vi "Main_v2.vi"(8 "error in (no error)":errorcluster) -> (0 "error out (no error)":errorcluster)   [LabVIEW 2019]
uses:
  controls/UI_Data_v2.ctl
  support/Copy of Message Queue/All Message Queues.ctl
  support/Copy of Message Queue/Message Cluster.ctl
  controls/MetaData_v2.ctl
  support/User Event - Stop/User Event - Stop.lvlib
  support/Copy of Message Queue/Copy of Message Queue.lvlib
  support/Message Queue/Message Queue.lvlib
panel:
  out "error out":errorcluster
  in  "UI Data":T1={"Measurements"=[], "Offsets"=[], "SSC"=[], "Message Queues"={"UI"=refnum, "Acquisition"=refnum, "Logging"=refnum, "Analyze"=refnum}, "MetaData"={"Operator Name"=enum."Operator Name", "Location"=enum."Location", "Sensor SN"="Sensor SN", "Cal Tube SN"="Cal Tube SN", "Comments"="Comments"}}
  in  "Stop":bool
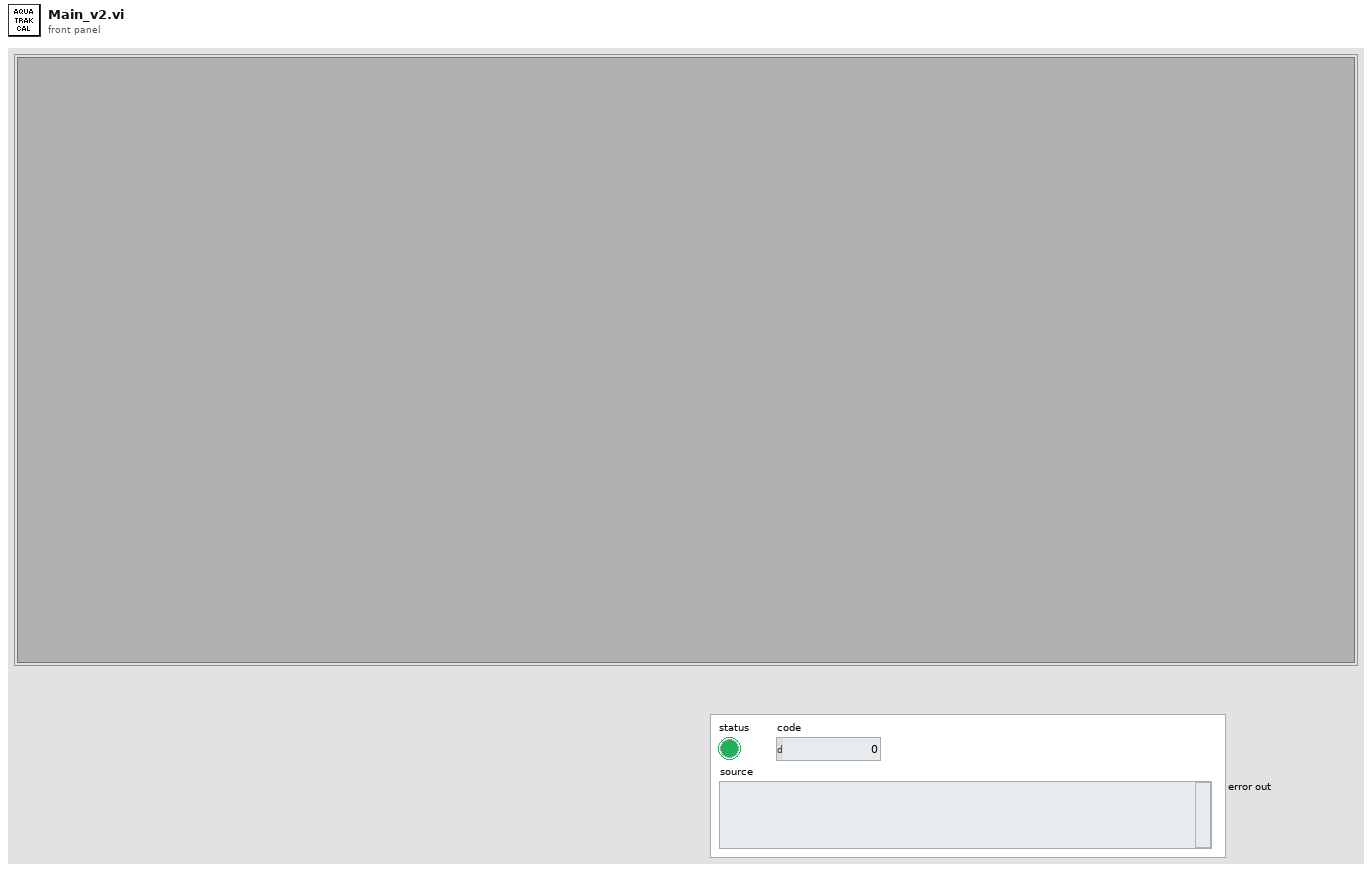
[diagram p1: front panel]
types:
  T1 = typedef "UI_Data_v2.ctl" = cluster{"Measurements":dbl[], "Offsets":dbl[], "SSC":dbl[], "Message Queues":T2, "MetaData":T3}
  T2 = typedef "Copy of Message Queue.lvlib/All Message Queues.ctl" = cluster{"UI":refnum<queue>, "Acquisition":refnum<queue>, "Logging":refnum<queue>, "Analyze":refnum<queue>}
  T3 = typedef "MetaData_v2.ctl" = cluster{"Operator Name":enum16{"Operator Name"}, "Location":enum16{"Location", "Chesapeake", "Silver Spring", "Seattle"}, "Sensor SN":string, "Cal Tube SN":string, "Comments":string}
  T4 = typedef "UserEvents_v2.ctl" = cluster{"User Event - Msg":refnum<user-event>, "User Event - Stop":refnum<user-event>}
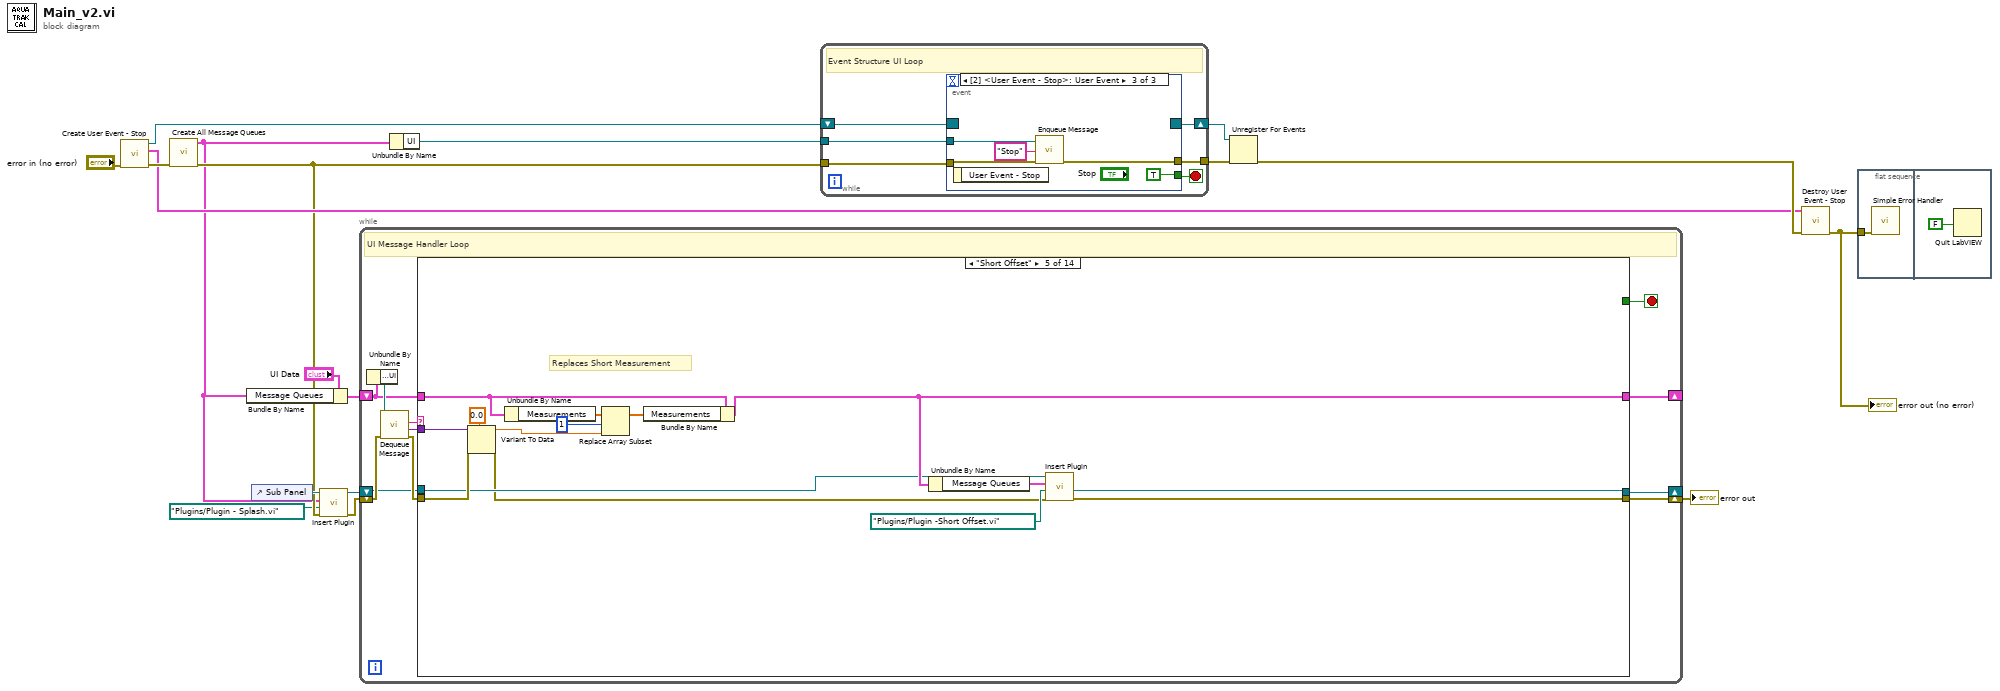
[diagram p0: block diagram]
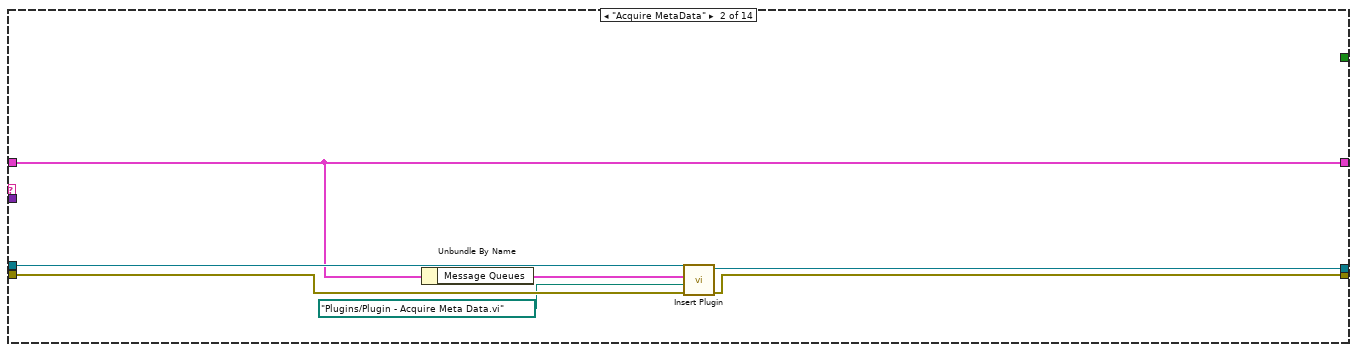
[diagram p3: hidden frame]
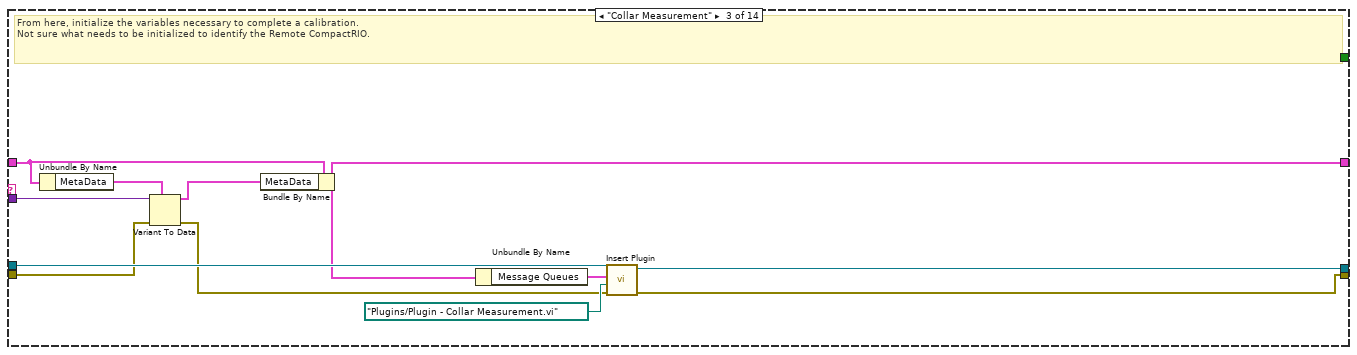
[diagram p4: hidden frame]
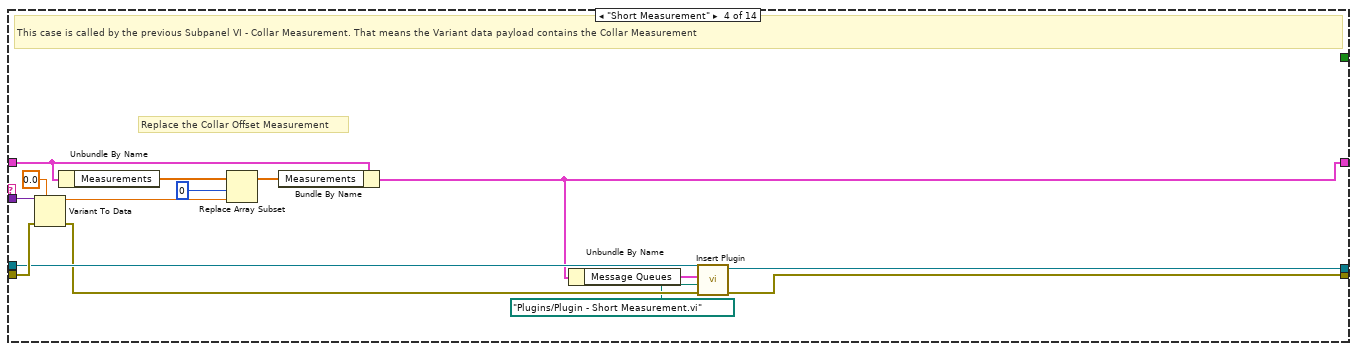
[diagram p5: hidden frame]
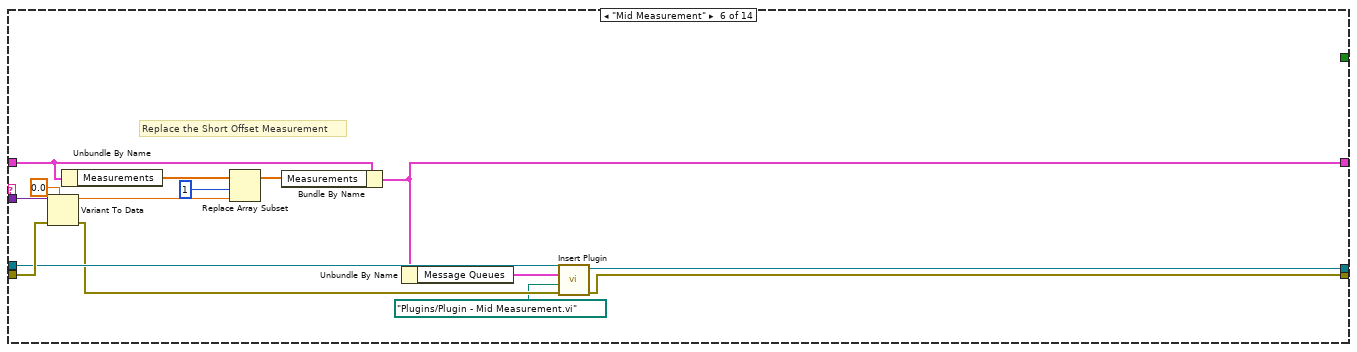
[diagram p6: hidden frame]
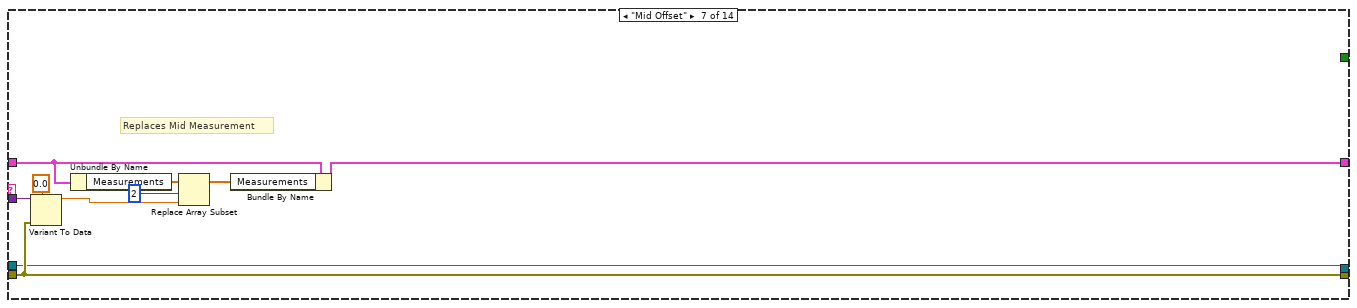
[diagram p7: hidden frame]
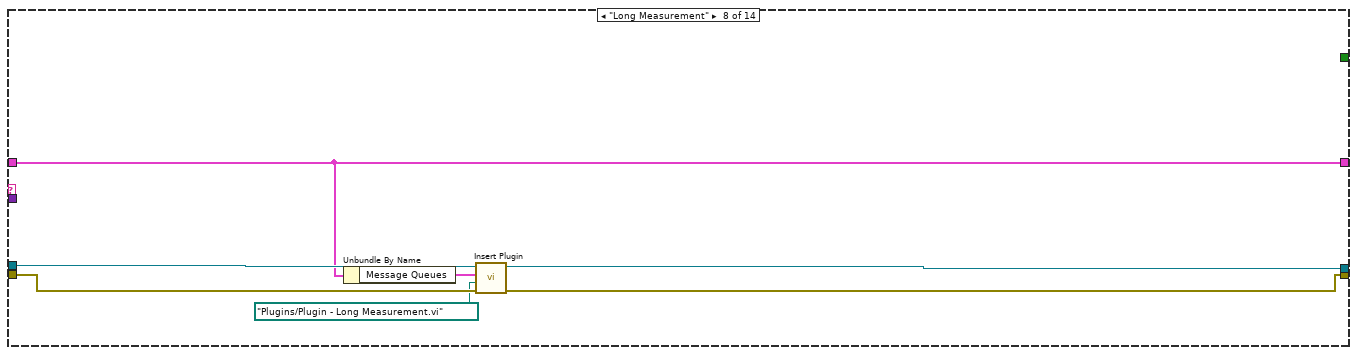
[diagram p8: hidden frame]
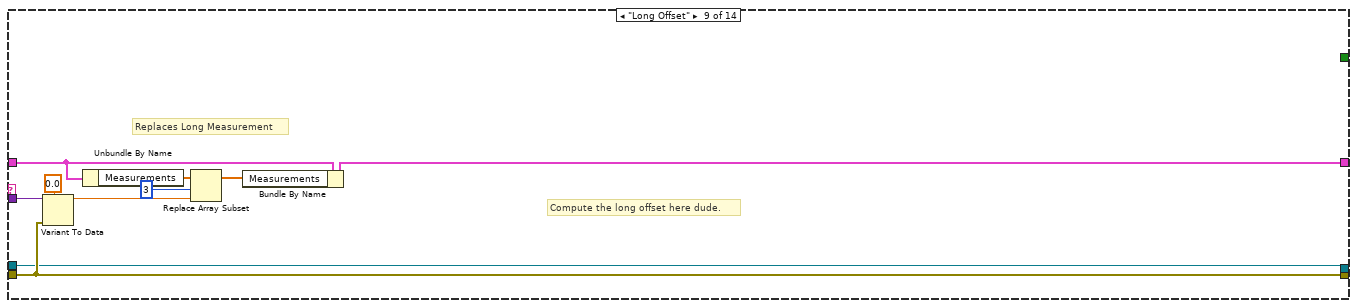
[diagram p9: hidden frame]
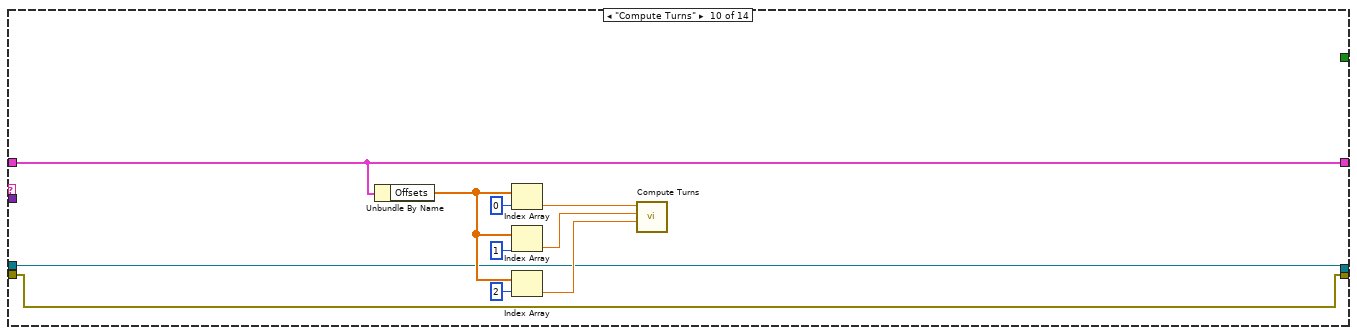
[diagram p10: hidden frame]
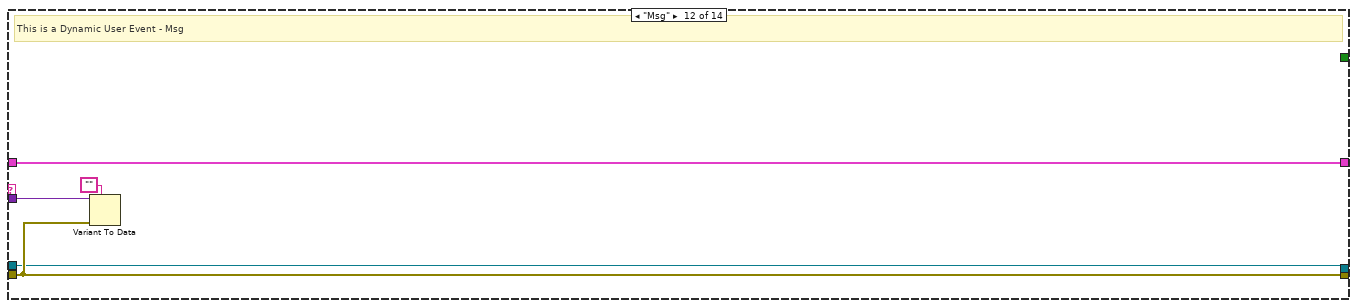
[diagram p12: hidden frame]
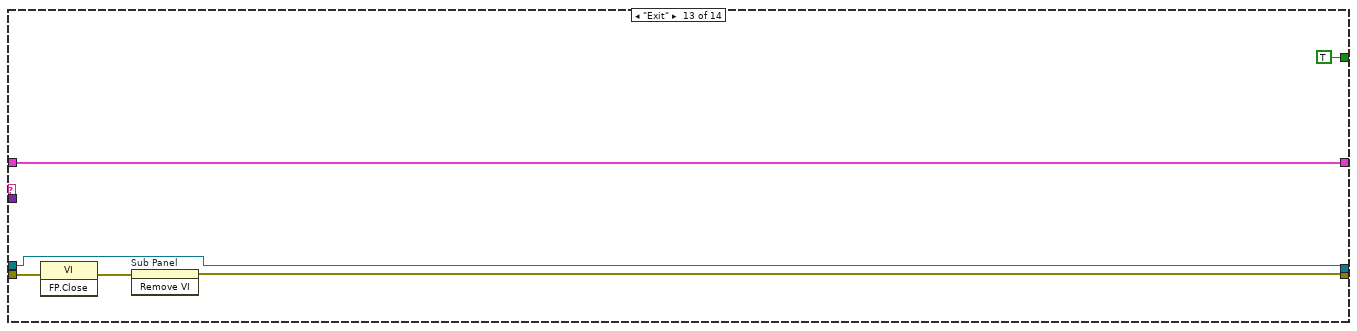
[diagram p13: hidden frame]
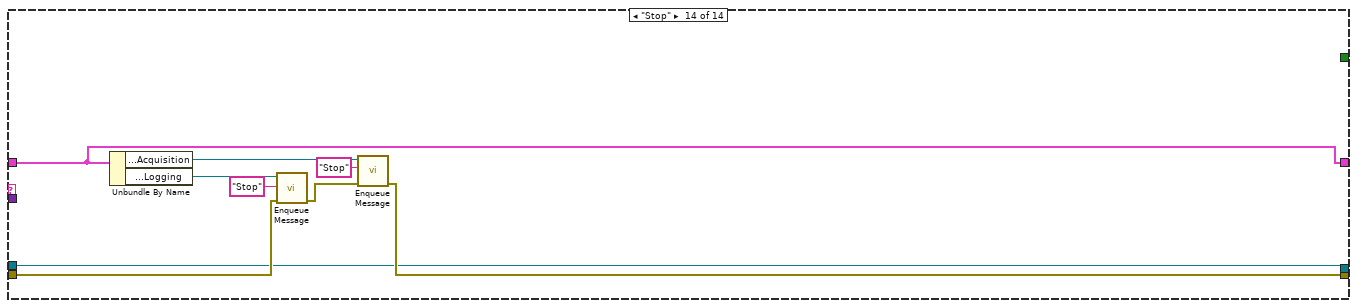
[diagram p14: hidden frame]
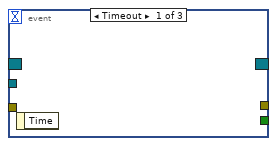
[diagram p15: hidden frame]
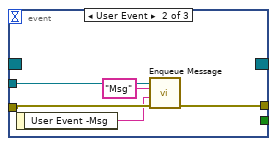
[diagram p16: hidden frame]
diagram:
  n1 = call "Create User Event - Stop.vi"("error in (no error)"="error in (no error)") -> ("error out"=w18:errorcluster, "User Events"=w8:T4, "Event Registration Refnum"=w17:refnum<event-registration>)  [unwired: 8 in]
  n2 = call "Create All Message Queues.vi"("error in (no error)"=w18) -> ("error out"=w5:errorcluster, "Message Queues out"=w1:T2)  [unwired: 9 in]
  n3 = Bundle By Name(cluster="UI Data", "Message Queues"=w1) -> (w9:T1)
  n4 = control-ref of="Sub Panel"() -> (w6:refnum<vi>)
  n5 = call "Insert Plugin.vi"("error in"=w5, "vi path"=path "Plugins/Plugin - Splash.vi", "Message Queues"=w1, "SubPanel in"=w6) -> ("error out"=w7:errorcluster, "SubPanel out"=w3:refnum<vi>)  [unwired: 6 in]
  n6 = while {
    shift-right: [w25] -> _
    shift-left: w9 -> [w26]
    shift-right: [w19] -> w2
    shift-left: w7 -> [w23]
    shift-right: [w20] -> _
    shift-left: w3 -> [w21]
    stop <- w24 stop-if-true
    # "UI Message Handler Loop"
    n7 = Unbundle By Name(w26) -> ("Message Queues.UI"=w29:refnum<queue>)
    n8 = call "Dequeue Message.vi"("error in (no error)"=w23, "Message Queue"=w29) -> ("error out"=w22:errorcluster, "Message Data"=w27:variant, "Message"=w28:string)  [unwired: 6 in, 1 out]
    n9 = case shown="\"Short Offset\"" w28 {
      tunnel: w27 -> [_ _ w44 w66 w75 w90 w99 _ w116 _ _ w141 _ _]
      tunnel: w26 -> [w32 w36 w46 w64 w76 w91 w101 w108 w117 w133 w136 w139 w146 w152]
      tunnel: [w32 w36 w45 w53 w73 w86 w100 w108 w118 w133 w136 w139 w146 w152] -> w25
      tunnel: [_ _ _ _ _ _ _ _ _ _ _ _ TRUE _] -> w24
      tunnel: w22 -> [w30 w38 w40 w59 w74 w89 w98 w110 w115 w124 w134 w138 w145 w151]
      tunnel: w21 -> [w31 w39 w51 w58 w69 w88 w97 w113 w114 w125 w135 w137 w142 w148]
      tunnel: [w30 w34 w50 w56 w67 w83 w98 w111 w115 w124 w134 w138 w143 w149] -> w19
      tunnel: [w31 w33 w49 w55 w70 w84 w97 w112 w114 w125 w135 w137 w142 w148] -> w20
      frame "Idle", Default {
        # "This Case structure keeps tabs of Present State."
      }
      frame "Acquire MetaData" {
        n10 = Unbundle By Name(w36) -> ("Message Queues"=w35:T2)
        n11 = call "Insert Plugin.vi"("error in"=w38, "vi path"=path "Plugins/Plugin - Acquire Meta Data.vi", "Message Queues"=w35, "SubPanel in"=w39) -> ("error out"=w34:errorcluster, "SubPanel out"=w33:refnum<vi>)  [unwired: 6 in]
      }
      frame "Collar Measurement" {
        # "From here, initialize the variables necessary to complete a calibration.\nNot sure what needs to be initialized to identify the Remote CompactRIO."
        n12 = Unbundle By Name(w46) -> ("MetaData"=w43:T3)
        n13 = Variant To Data(error in=w40, type=w43, Variant=w44) -> (data=w42:T3, error out=w41:errorcluster)
        n14 = Bundle By Name(cluster=w46, "MetaData"=w42) -> (w45:T1)
        n15 = Unbundle By Name(w45) -> ("Message Queues"=w47:T2)
        n16 = call "Insert Plugin.vi"("error in"=w41, "vi path"=path "Plugins/Plugin - Collar Measurement.vi", "Message Queues"=w47, "SubPanel in"=w51) -> ("error out"=w50:errorcluster, "SubPanel out"=w49:refnum<vi>)  [unwired: 6 in]
      }
      frame "Short Measurement" {
        # "Replace the Collar Offset Measurement"
        # "This case is called by the previous Subpanel VI - Collar Measurement. That means the Variant data payload contains the Collar Measurement"
        n17 = Variant To Data(error in=w59, type=0.0 ("Measurements"), Variant=w66) -> (data=w60:dbl, error out=w57:errorcluster)
        n18 = Unbundle By Name(w64) -> ("Measurements"=w62:dbl[])
        n19 = Replace Array Subset(array=w62, new element=w60, index=0) -> (w63:dbl[])
        n20 = Bundle By Name(cluster=w64, "Measurements"=w63) -> (w53:T1)
        n21 = Unbundle By Name(w53) -> ("Message Queues"=w52:T2)
        n22 = call "Insert Plugin.vi"("error in"=w57, "vi path"=path "Plugins/Plugin - Short Measurement.vi", "Message Queues"=w52, "SubPanel in"=w58) -> ("error out"=w56:errorcluster, "SubPanel out"=w55:refnum<vi>)  [unwired: 6 in]
      }
      frame "Short Offset" {
        # "Replaces Short Measurement"
        n23 = Variant To Data(error in=w74, type=0.0 ("Measurements"), Variant=w75) -> (data=w77:dbl, error out=w68:errorcluster)
        n24 = Unbundle By Name(w76) -> ("Measurements"=w79:dbl[])
        n25 = Replace Array Subset(array=w79, new element=w77, index=1) -> (w80:dbl[])
        n26 = Bundle By Name(cluster=w76, "Measurements"=w80) -> (w73:T1)
        n27 = Unbundle By Name(w73) -> ("Message Queues"=w72:T2)
        n28 = call "Insert Plugin.vi"("error in"=w68, "vi path"=path "Plugins/Plugin -Short Offset.vi", "Message Queues"=w72, "SubPanel in"=w69) -> ("error out"=w67:errorcluster, "SubPanel out"=w70:refnum<vi>)  [unwired: 6 in]
      }
      frame "Mid Measurement" {
        # "Replace the Short Offset Measurement"
        n29 = Variant To Data(error in=w89, type=0.0 ("Measurements"), Variant=w90) -> (data=w92:dbl, error out=w87:errorcluster)
        n30 = Unbundle By Name(w91) -> ("Measurements"=w94:dbl[])
        n31 = Replace Array Subset(array=w94, new element=w92, index=1) -> (w95:dbl[])
        n32 = Bundle By Name(cluster=w91, "Measurements"=w95) -> (w86:T1)
        n33 = Unbundle By Name(w86) -> ("Message Queues"=w85:T2)
        n34 = call "Insert Plugin.vi"("error in"=w87, "vi path"=path "Plugins/Plugin - Mid Measurement.vi", "Message Queues"=w85, "SubPanel in"=w88) -> ("error out"=w83:errorcluster, "SubPanel out"=w84:refnum<vi>)  [unwired: 6 in]
      }
      frame "Mid Offset" {
        # "Replaces Mid Measurement"
        n35 = Variant To Data(error in=w98, type=0.0 ("Measurements"), Variant=w99) -> (data=w102:dbl)  [unwired: 1 out]
        n36 = Unbundle By Name(w101) -> ("Measurements"=w104:dbl[])
        n37 = Replace Array Subset(array=w104, new element=w102, index=2) -> (w105:dbl[])
        n38 = Bundle By Name(cluster=w101, "Measurements"=w105) -> (w100:T1)
      }
      frame "Long Measurement" {
        n39 = Unbundle By Name(w108) -> ("Message Queues"=w107:T2)
        n40 = call "Insert Plugin.vi"("error in"=w110, "vi path"=path "Plugins/Plugin - Long Measurement.vi", "Message Queues"=w107, "SubPanel in"=w113) -> ("error out"=w111:errorcluster, "SubPanel out"=w112:refnum<vi>)  [unwired: 6 in]
      }
      frame "Long Offset" {
        # "Compute the long offset here dude."
        # "Replaces Long Measurement"
        n41 = Variant To Data(error in=w115, type=0.0 ("Measurements"), Variant=w116) -> (data=w119:dbl)  [unwired: 1 out]
        n42 = Unbundle By Name(w117) -> ("Measurements"=w121:dbl[])
        n43 = Replace Array Subset(array=w121, new element=w119, index=3) -> (w122:dbl[])
        n44 = Bundle By Name(cluster=w117, "Measurements"=w122) -> (w118:T1)
      }
      frame "Compute Turns" {
        n45 = Unbundle By Name(w133) -> ("Offsets"=w130:dbl[])
        n46 = Index Array(array=w130, index=0) -> (element=w132:dbl)
        n47 = Index Array(array=w130, index=1) -> (element=w131:dbl)
        n48 = Index Array(array=w130, index=2) -> (element=w129:dbl)
        n49 = call "Compute Turns.vi"("Long Offset"=w129, "Mid Offset"=w131, "Short Offset"=w132) -> ()  [unwired: 8 in, 1 out]
      }
      frame "Compute Final Offset" {
      }
      frame "Msg" {
        # "This is a Dynamic User Event - Msg"
        n50 = Variant To Data(error in=w138, type="", Variant=w141) -> ()  [unwired: 2 out]
      }
      frame "Exit" {
        n51 = invoke class="VI" method="FP.Close"(error in=w145) -> (error out=w144:errorcluster)  [unwired: 2 in, 2 out]
        n52 = invoke on="Sub Panel" class="SubPnl" method="Remove VI"(error in=w144) -> (error out=w143:errorcluster)  [unwired: 2 in, 2 out]
      }
      frame "Stop" {
        n53 = Unbundle By Name(w152) -> ("Message Queues.Acquisition"=w153:refnum<queue>, "Message Queues.Logging"=w155:refnum<queue>)
        n54 = call "Enqueue Message.vi"("error in (no error)"=w151, "Message"="Stop", "Message Queue"=w155) -> ("error out"=w150:errorcluster)  [unwired: 7 in, 1 out]
        n55 = call "Enqueue Message.vi"("error in (no error)"=w150, "Message"="Stop", "Message Queue"=w153) -> ("error out"=w149:errorcluster)  [unwired: 7 in, 1 out]
      }
    }
  }
  "error out" <- w2
  n56 = Unbundle By Name(w1) -> ("UI"=w13:refnum<queue>)
  n57 = while {
    shift-right: [w160] -> w15
    shift-left: w17 -> [w161]
    tunnel: [w159] -> w14
    tunnel: w13 -> [w158]
    tunnel: w5 -> [w157]
    stop <- w162 stop-if-true
    # "Event Structure UI Loop"
    n58 = event shown="[2] <User Event - Stop>: User Event" {
      selector: w161 -> [_ _ _]
      dyn-events: [_ _ _] -> w160
      timeout: _ -> [_ _ _]
      tunnel: [_ _ TRUE ("Stop")] -> w162
      tunnel: [_ w164 w171] -> w159
      tunnel: w158 -> [_ w166 w170]
      tunnel: w157 -> [_ w165 w169]
      event Timeout {
        n59 = event-data() -> ()  [unwired: 1 in, 1 out]
      }
      event User Event {
        n60 = event-data() -> ("User Event -Msg"=w163:string)  [unwired: 1 in]
        n61 = call "Enqueue Message.vi"("error in (no error)"=w165, "Message Data"=w163, "Message"="Msg", "Message Queue"=w166) -> ("error out"=w164:errorcluster)  [unwired: 6 in, 1 out]
      }
      event User Event {
        n62 = event-data() -> ()  [unwired: 1 in, 1 out]
        n63 = call "Enqueue Message.vi"("error in (no error)"=w169, "Message"="Stop", "Message Queue"=w170) -> ("error out"=w171:errorcluster)  [unwired: 7 in, 1 out]
      }
    }
  }
  n64 = Unregister For Events(event registration refnum=w15, error in=w14) -> (error out=w16:errorcluster)
  n65 = call "Destroy User Event - Stop.vi"("error in (no error)"=w16, "User Events in"=w8) -> ("error out"=w11:errorcluster)  [unwired: 9 in]
  "error out (no error)" <- w11
  n66 = flat-sequence {
    tunnel: w11 -> [w173]
    frame #0 {
      n67 = call <vilib>:"Simple Error Handler.vi"("error in (no error)"=w173) -> ()  [unwired: 4 in, 5 out]
    }
    frame #1 {
      n68 = Quit LabVIEW(quit? (T)=FALSE) -> ()
    }
  }
